vi "add,sub,mult 2.vi"() -> ()   [LabVIEW 2025]
panel:
  in  "b":dbl
  out "c":dbl
  in  "a":dbl
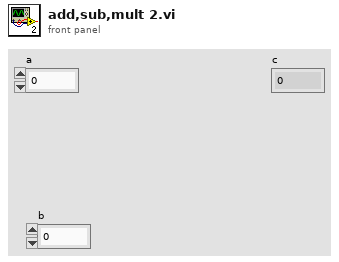
[diagram p1: front panel]
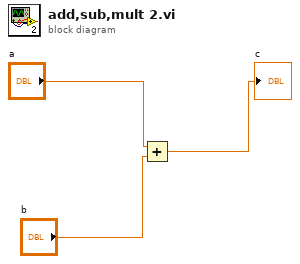
[diagram p0: block diagram]
diagram:
  n1 = Add(x="a", y="b") -> (x+y=→"c":dbl)
